vi "Launch Nested.vi"(6 "Wait to Start (F)":bool, 7 "API Type (Base)":refnum<class "Actor API.lvclass">, 8 "error in (no error)":errorcluster, 10 "Nested Actor":refnum<class "Actor.lvclass">, 11 "Actor in":refnum<class "Actor.lvclass">) -> (0 "error out":errorcluster, 2 "Nested API":refnum<class "Actor API.lvclass">, 3 "Actor out":refnum<class "Actor.lvclass">)   [LabVIEW 2020, in "Artifex.lvlib" / "Actor.lvclass"]
uses:
  Actor.lvclass
  Actor Proxy/Actor API.lvclass
panel:
  in  "Auto Stop (T)":bool=TRUE
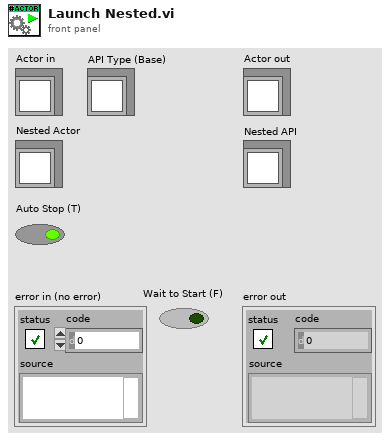
[diagram p1: front panel]
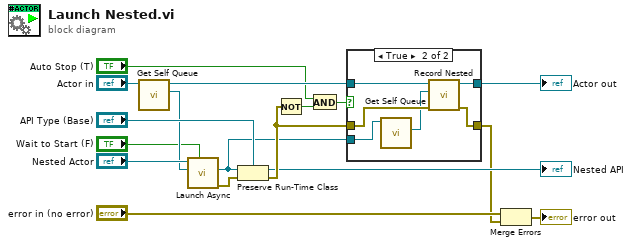
[diagram p0: block diagram]
diagram:
  n1 = call "Get Self Queue.vi"("Actor in"="Actor in") -> ("Self Queue"=w2:refnum<class "Priority Message Queue.lvclass">, "Actor out"=w12:refnum<class "Actor.lvclass">)  [unwired: 9 in]
  n2 = call "Launch Async.vi"("Wait to Start"="Wait to Start (F)", "Caller Queue"=w2, "Actor in"="Nested Actor") -> ("error out"=w14:errorcluster, "Actor API"=w8:refnum<class "Actor API.lvclass">)  [unwired: 7 in]
  n3 = Preserve Run-Time Class(object in=w8, error in=w14, 2:"API Type (Base)") -> (object out=→"Nested API":refnum<class "Actor API.lvclass">, error out=w17:errorcluster)
  n4 = Not(x=w17) -> (.not. x?=w11:bool)
  n5 = And(x="Auto Stop (T)", y=w11) -> (x .and. y?=w9:bool)
  n6 = case shown="True" w9 {
    tunnel: w12 -> [w19 w23]
    tunnel: w17 -> [w18 w25]
    tunnel: w8 -> [_ w24]
    tunnel: [w18 w21] -> w5
    tunnel: [w19 w20] -> w7
    frame False {
    }
    frame True {
      n7 = call "Get Self Queue.vi"("Actor API in"=w24) -> ("Self Queue"=w22:refnum<class "Priority Message Queue.lvclass">)  [unwired: 8 in, 2 out]
      n8 = call "Record Nested.vi"("error in (no error)"=w25, "Nested Queue"=w22, "Actor in"=w23) -> ("error out"=w21:errorcluster, "Actor out"=w20:refnum<class "Actor.lvclass">)  [unwired: 7 in]
    }
  }
  "Actor out" <- w7
  n9 = Merge Errors("error in (no error)", w5) -> (→"error out":errorcluster)
